vi "Instr_InitObject.vi"(8 "error in (no error)":errorcluster, 9 "Instrument Configuration":variant, 10 "GPIB Address":string, 11 "KE2000 in":refnum<class "KE2000.lvclass">) -> (0 "error out":errorcluster, 3 "KE2000 out":refnum<class "KE2000.lvclass">)   [LabVIEW 2018, in "KE2000.lvclass"]
uses:
  KE2000.lvclass
  InstrumentSetup.vi
  KE2000_CommandsGlobal.vi
  MultimeterControl.lvclass
  InstrControl.lvclass
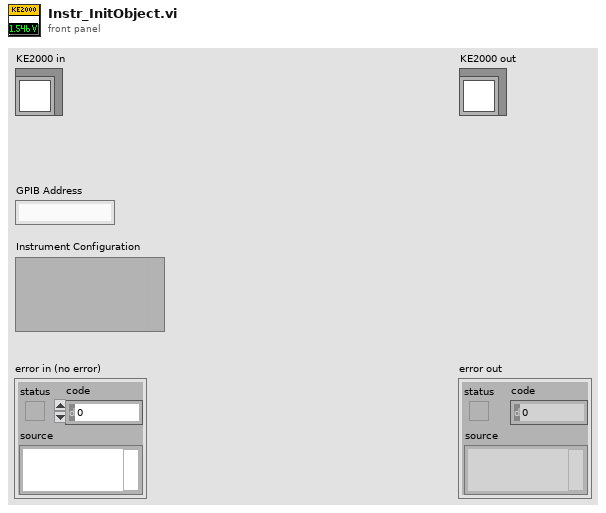
[diagram p1: front panel]
types:
  T1 = cluster{"Range":u16, "Range Value":dbl, "Function":u16}
  T2 = cluster{"Instrument name":string, "Command \"Reset\"":string, "Command \"Initialise\"":string, "Command \"Read Data\"":string}
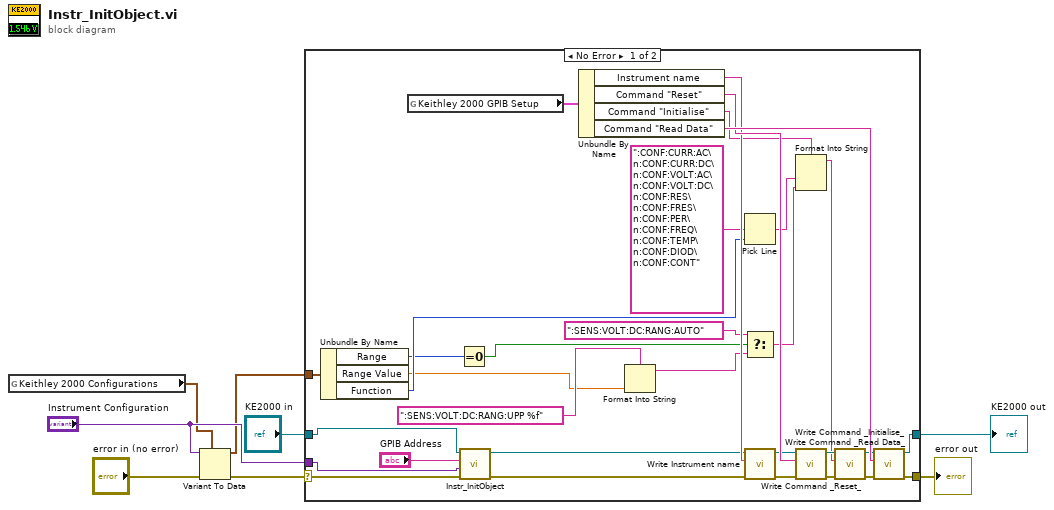
[diagram p0: block diagram]
diagram:
  n1 = global read "InstrumentSetup.vi" "Keithley 2000 Configurations"() -> (w2:T1)
  n2 = Variant To Data(error in="error in (no error)", type=w2, Variant="Instrument Configuration") -> (data=w1:T1, error out=w4:errorcluster)
  n3 = case shown="No Error" w4 {
    selector: w4 -> [w15 w41]
    tunnel: [w35 w41] -> w8
    tunnel: "KE2000 in" -> [w17 w40]
    tunnel: [w32 w40] -> w6
    tunnel: "Instrument Configuration" -> [w11 _]
    tunnel: w1 -> [w9 _]
    frame No Error {
      n4 = Unbundle By Name(w9) -> ("Range"=w25:u16, "Range Value"=w23:dbl, "Function"=w28:u16)
      n5 = global read "KE2000_CommandsGlobal.vi" "Keithley 2000 GPIB Setup"() -> (w10:T2)
      n6 = Equal To 0?(x=w25) -> (x = 0?=w26:bool)
      n7 = call-parent "Instr_InitObject.vi"("error in (no error)"=w15, "Instrument Configuration"=w11, "GPIB Address"="GPIB Address", "MultimeterControl in"=w17) -> ("error out"=w14:errorcluster, "MultimeterControl out"=w16:refnum<class "KE2000.lvclass">)  [unwired: 6 in]
      n8 = Unbundle By Name(w10) -> ("Instrument name"=w31:string, "Command \"Reset\""=w38:string, "Command \"Initialise\""=w30:string, "Command \"Read Data\""=w39:string)
      n9 = Format Into String(format string=":SENS:VOLT:DC:RANG:UPP %f", w23) -> (resulting string=w22:string)  [unwired: 2 in, 1 out]
      n10 = Pick Line(multi-line string=":CONF:CURR:AC\n:CONF:CURR:DC\n:CONF:VOLT:AC\n:CONF:VOLT:DC\n:CONF:RES\n:CONF:FRES\n:CONF:PER\n:CONF:FREQ\n:CONF:TEMP\n:CONF:DIOD\n:CONF:CONT", line index=w28) -> (output string=w27:string)  [unwired: 1 in]
      n11 = Select(t=":SENS:VOLT:DC:RANG:AUTO", s=w26, f=w22) -> (s? t:f=w20:string)
      n12 = call-dynamic "Write Instrument name.vi"("error in (no error)"=w14, "Instrument name"=w31, "InstControl in"=w16) -> ("error out"=w12:errorcluster, "InstControl out"=w13:refnum<class "KE2000.lvclass">)  [unwired: 7 in]
      n13 = Format Into String(format string=w30, w27, w20) -> (resulting string=w19:string)  [unwired: 2 in, 1 out]
      n14 = call-dynamic "Write Command _Reset_.vi"("error in (no error)"=w12, "Command \"Reset\""=w38, "MultimeterControl in"=w13) -> ("error out"=w37:errorcluster, "MultimeterControl out"=w34:refnum<class "KE2000.lvclass">)  [unwired: 7 in]
      n15 = call-dynamic "Write Command _Initialise_.vi"("error in (no error)"=w37, "Command \"Initialise\""=w19, "MultimeterControl in"=w34) -> ("error out"=w36:errorcluster, "MultimeterControl out"=w33:refnum<class "KE2000.lvclass">)  [unwired: 7 in]
      n16 = call-dynamic "Write Command _Read Data_.vi"("error in (no error)"=w36, "Command \"Read Data\""=w39, "MultimeterControl in"=w33) -> ("error out"=w35:errorcluster, "MultimeterControl out"=w32:refnum<class "KE2000.lvclass">)  [unwired: 7 in]
    }
    frame Error {
    }
  }
  "error out" <- w8
  "KE2000 out" <- w6
